vi "Calculate Counter And Protections.vi"(8 "error in (no error)":errorcluster, 9 "timeout ms":i32=100, 10 "Async Settings":T1={"Priority"=100, "CAN Session"="", "Frame Count"=0, "Frames"=[], "FPGA Session"=0, "Incoming Frame Session"="", "Incoming Session Invalid"=FALSE, "Incoming Frames"=[], "Signal Values"=[], "Incoming Signal Info"={"Signal.PrevData"=[], "Signal Names"=[], "Signal Settings Out"=[]}} {"Incoming Signal Info"."Signal Settings Out"."Protection Configuration"."CRC Channels"."Data Type" items=["Signed", "Unsigned", "IEEE Float"]; "Incoming Frames"."Protection Configurations"."CRC Channels"."Data Type" items=["Signed", "Unsigned", "IEEE Float"]; "Frames"."Protection Configurations"."CRC Channels"."Data Type" items=["Signed", "Unsigned", "IEEE Float"]}, 11 "Data Refs":T13) -> (0 "error out":errorcluster, 2 "Async Settings":T1={"Priority"=100, "CAN Session"="", "Frame Count"=0, "Frames"=[], "FPGA Session"=0, "Incoming Frame Session"="", "Incoming Session Invalid"=FALSE, "Incoming Frames"=[], "Signal Values"=[], "Incoming Signal Info"={"Signal.PrevData"=[], "Signal Names"=[], "Signal Settings Out"=[]}} {"Incoming Signal Info"."Signal Settings Out"."Protection Configuration"."CRC Channels"."Data Type" items=["Signed", "Unsigned", "IEEE Float"]; "Incoming Frames"."Protection Configurations"."CRC Channels"."Data Type" items=["Signed", "Unsigned", "IEEE Float"]; "Frames"."Protection Configurations"."CRC Channels"."Data Type" items=["Signed", "Unsigned", "IEEE Float"]})   [LabVIEW 2015, in "Protection and Counter Addon Engine.lvlib"]
uses:
  Protection and Counter Addon Engine.lvlib
  Types/RT Async Engine Variables.ctl
  SubModules/Frame Protection Support/Source/Engine/Types/RT Frame Settings.ctl
  SubModules/Frame Protection Support/Source/Shared/Types/Exported Frame Type.ctl
  SubModules/Frame Protection Support/Source/Engine/Types/RT Protection Configuration.ctl
  SubModules/Frame Protection Support/Source/Shared/Types/Protection Type.ctl
  SubModules/Frame Protection Support/Source/Shared/Types/XNET Signal Configuration.ctl
  SubModules/Frame Protection Support/Source/Shared/Types/Exported Counter Settings.ctl
  SubModules/Frame Protection Support/Source/Shared/Types/Exported Event Trigger Type.ctl
  SubModules/Frame Protection Support/Source/Shared/Types/Exported Frame Settings.ctl
  SubModules/Frame Protection Support/Source/Shared/Types/Exported Protection Settings.ctl
  SubModules/Frame Protection Support/Source/Shared/Types/RT_Incoming_Signal_Info.ctl
  SubModules/Frame Protection Support/Source/Shared/Types/RT Exported Signal Settings.ctl
  Types/RT Data References.ctl
  <vilib>/NI/NIVS Inline Async API/_Data Access Engine/Data Access Engine/Types/Write.DVR.ctl
  <vilib>/NI/NIVS Inline Async API/_Data Access Engine/Access Type Classes/Write/Write.lvclass
  <vilib>/NI/NIVS Inline Async API/_Data Access Engine/Data Access Engine/Types/Read.DVR.ctl
  <vilib>/NI/NIVS Inline Async API/_Data Access Engine/Access Type Classes/Read/Read.lvclass
  <vilib>/NI/NIVS Inline Async API/_Data Access Engine/Access Type Classes/Read/Read.lvclass/Read.ctl
  <vilib>/NI/NIVS Inline Async API/_Data Access Engine/Access Type Classes/Write/Write.lvclass/Write.ctl
  <vilib>/NI/NIVS Inline Async API/_Data Access Engine/Data Access Engine/Methods/Write.Data.vi
  <vilib>/NI/NIVS Inline Async API/_Data Access Engine/Access Type Classes/Write/Write.ProcessData.vi
  <vilib>/NI/NIVS Inline Async API/_Data Access Engine/Data Access Engine/Methods/Read.Data.Detect.vi
  <vilib>/NI/NIVS Inline Async API/_Data Access Engine/Data Access Engine/Methods/Write.Data.Buffer.vi
  SubModules/Frame Protection Support/Source/Engine/SubVIs/Determine Transmission.vi
  SubModules/Frame Protection Support/Source/Engine/SubVIs/Determine Periodic.vi
  <vilib>/NI/NIVS Inline Async API/_Data Access Engine/Data Access Engine/Methods/Write.Data.Commit.vi
  <vilib>/NI/NIVS Inline Async API/_Data Access Engine/Access Type Classes/Read/Read.ProcessData.Detect.vi
  <vilib>/NI/NIVS Inline Async API/_Data Access Engine/Access Type Classes/Write/Write.Buffer.vi
  <vilib>/NI/NIVS Inline Async API/_Data Access Engine/Access Type Classes/Write/Write.Commit.vi
  <vilib>/xnet/xnet.llb/XNET Write (Frame CAN).vi
  <vilib>/xnet/xnet.llb/XNET Convert.vi
  <vilib>/xnet/xnet.llb/XNET Convert (Signal to Frame CAN).vi
  <vilib>/xnet/xnet.llb/XNET Convert (Signal to Frame Raw).vi
  <vilib>/NI/NIVS Inline Async API/_Data Access Engine/Data Access Engine/Data Access Engine.lvclass
  SubModules/Frame Protection Support/Source/Engine/Protection and Counter Support Engine.lvlib
  SubModules/Frame Protection Support/Source/Shared/Protection and Counter Support Shared.lvlib
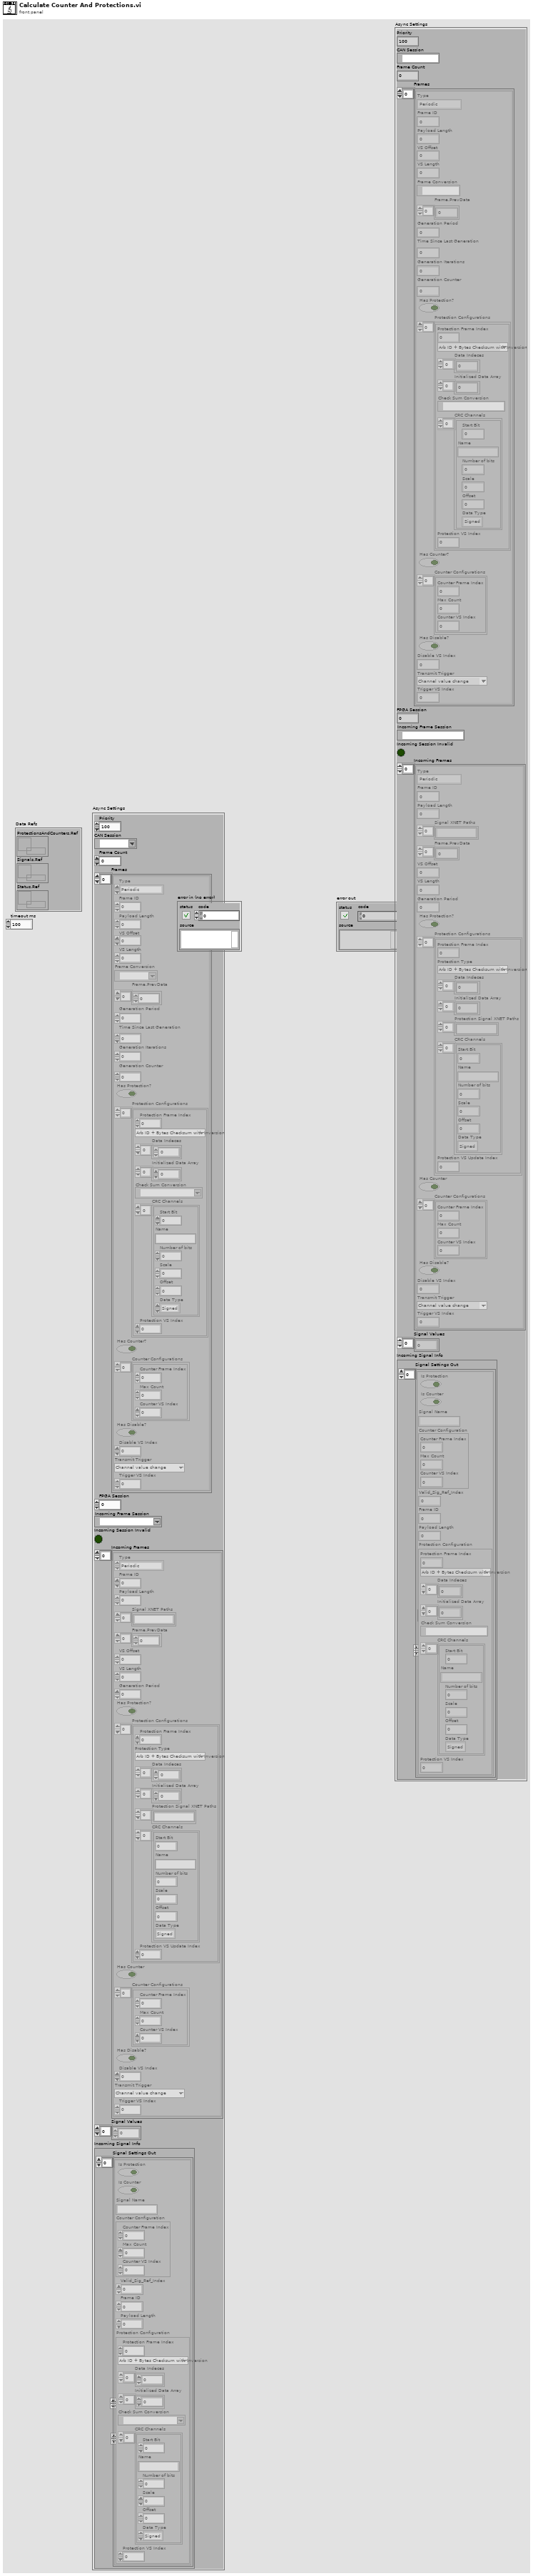
[diagram p1: front panel]
types:
  T1 = typedef "Protection and Counter Addon Engine.lvlib/RT Async Engine Variables.ctl" = cluster{"Priority":i32, "CAN Session":refnum<k21>, "Frame Count":i32, "Frames":T2[], "FPGA Session":u32, "Incoming Frame Session":refnum<k21>, "Incoming Session Invalid":bool, "Incoming Frames":T9[], "Signal Values":dbl[], "Incoming Signal Info":T11}
  T2 = typedef "Protection and Counter Support Engine.lvlib/RT Frame Settings.ctl" = cluster{"Type":T3, "Frame ID":u32, "Payload Length":u32, "VS Offset":i32, "VS Length":i32, "Frame Conversion":refnum<k21>, "Frame.PrevData":dbl[], "Generation Period":u32, "Time Since Last Generation":u32, "Generation Iterations":u32, "Generation Counter":u32, "Has Protection?":bool, "Protection Configurations":T4[], "Has Counter?":bool, "Counter Configurations":T7[], "Has Disable?":bool, "Disable VS Index":i32, "Transmit Trigger":T8, "Trigger VS Index":i32}
  T3 = typedef "Protection and Counter Support Shared.lvlib/Exported Frame Type.ctl" = enum16{"Periodic", "Event", "Periodic/Event"}
  T4 = typedef "Protection and Counter Support Engine.lvlib/RT Protection Configuration.ctl" = cluster{"Protection Frame Index":i32, "Protection Type":T5, "Data Indeces":i32[], "Initialized Data Array":dbl[], "Check Sum Conversion":refnum<k21>, "CRC Channels":T6[], "Protection VS Index":i32}
  T5 = typedef "Protection and Counter Support Shared.lvlib/Protection Type.ctl" = enum16{"Arb ID + Bytes Checksum with Inversion", "Arb ID + Bytes CRC with Inversion", "Reversed Raw Signal Checksum with Inversion"}
  T6 = typedef "Protection and Counter Support Shared.lvlib/XNET Signal Configuration.ctl" = cluster{"Start Bit":i32, "Name":string, "Number of bits":i32, "Scale":dbl, "Offset":dbl, "Data Type":u32}
  T7 = typedef "Protection and Counter Support Shared.lvlib/Exported Counter Settings.ctl" = cluster{"Counter Frame Index":i32, "Max Count":dbl, "Counter VS Index":i32}
  T8 = typedef "Protection and Counter Support Shared.lvlib/Exported Event Trigger Type.ctl" = enum16{"Channel value change", "Trigger channel (not zero)", "Channel value change or trigger channel (not zero)", "Trigger channel (any value change)", "Channel value change or trigger channel (any value change)"}
  T9 = typedef "Protection and Counter Support Shared.lvlib/Exported Frame Settings.ctl" = cluster{"Type":T3, "Frame ID":u32, "Payload Length":u32, "Signal XNET Paths":string[], "Frame.PrevData":dbl[], "VS Offset":i32, "VS Length":i32, "Generation Period":u32, "Has Protection?":bool, "Protection Configurations":T10[], "Has Counter":bool, "Counter Configurations":T7[], "Has Disable?":bool, "Disable VS Index":i32, "Transmit Trigger":T8, "Trigger VS Index":i32}
  T10 = typedef "Protection and Counter Support Shared.lvlib/Exported Protection Settings.ctl" = cluster{"Protection Frame Index":i32, "Protection Type":T5, "Data Indeces":i32[], "Initialized Data Array":dbl[], "Protection Signal XNET Paths":string[], "CRC Channels":T6[], "Protection VS Update Index":i32}
  T11 = typedef "Protection and Counter Support Shared.lvlib/RT_Incoming_Signal_Info.ctl" = cluster{"Signal.PrevData":dbl[], "Signal Names":string[], "Signal Settings Out":T12[]}
  T12 = typedef "Protection and Counter Support Shared.lvlib/RT Exported Signal Settings.ctl" = cluster{"Is Protection":bool, "Is Counter":bool, "Signal Name":string, "Counter Configuration":T7, "Valid_Sig_Ref_Index":i32, "Frame ID":u32, "Payload Length":u32, "Protection Configuration":T4}
  T13 = typedef "Protection and Counter Addon Engine.lvlib/RT Data References.ctl" = cluster{"ProtectionsAndCounters.Ref":T14, "Signals.Ref":T15, "Status.Ref":T14}
  T14 = typedef "Data Access Engine.lvlib/Data Access Engine.lvclass/Write.DVR.ctl" = refnum<data-value>
  T15 = typedef "Data Access Engine.lvlib/Data Access Engine.lvclass/Read.DVR.ctl" = refnum<data-value>
  T16 = typedef "XNET Frame CAN.ctl" = cluster{"timestamp":timestamp, "payload":u8[], "identifier":u32, "type":T17, "extended?":bool, "echo?":bool}
  T17 = typedef "XNET Frame Type CAN.ctl" = u8
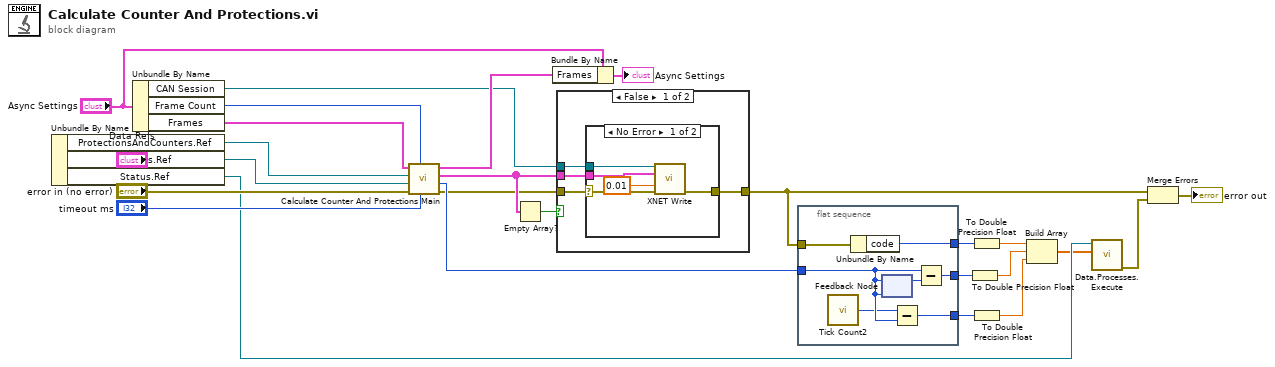
[diagram p0: block diagram]
diagram:
  n1 = Unbundle By Name("Data Refs") -> ("ProtectionsAndCounters.Ref"=w1:T14, "Signals.Ref"=w21:T15, "Status.Ref"=w19:T14)
  n2 = Unbundle By Name("Async Settings") -> ("CAN Session"=w6:refnum<k21>, "Frame Count"=w23:i32, "Frames"=w2:T2[])
  n3 = call "Calculate Counter And Protections Main.vi"("timeout ms"="timeout ms", "Frame Count"=w23, "error in (no error)"="error in (no error)", "Signals"=w21, "Protections"=w1, "Frames in"=w2) -> ("error out"=w5:errorcluster, "Tick Count(uSec)"=w20:u32, "Frames"=w9:T16[], "Frames out"=w11:T2[])  [unwired: 2 in]
  n4 = Empty Array?(array=w9) -> (empty?=w8:bool)
  n5 = Bundle By Name(cluster="Async Settings", "Frames"=w11) -> (→"Async Settings":T1)
  n6 = case shown="False" w8 {
    tunnel: w5 -> [w30 w37]
    tunnel: [w29 w37] -> w4
    tunnel: w6 -> [w28 _]
    tunnel: w9 -> [w27 _]
    frame False {
      n7 = case shown="No Error" w30 {
        selector: w30 -> [w32 w36]
        tunnel: w27 -> [w35 _]
        tunnel: [w34 w36] -> w29
        tunnel: w28 -> [w33 _]
        frame No Error {
          n8 = call-poly <vilib>:"XNET Write.vi"("session in"=w33, "data"=w35, "timeout (10)"=0.01, "error in (no error)"=w32) -> ("error out"=w34:errorcluster)  [unwired: 10 in, 1 out]
        }
        frame Error {
        }
      }
    }
    frame True {
    }
  }
  n9 = flat-sequence {
    tunnel: w20 -> [w44]
    tunnel: [w43] -> w18
    tunnel: [w42] -> w15
    tunnel: w4 -> [w39]
    tunnel: [w38] -> w7
    frame #0 {
      n10 = call "Tick Count2"() -> ("Tick Count(uSec)"=w41:u32)
      n11 = Unbundle By Name(w39) -> ("code"=w38:i32)
      n12 = feedback #1(w44) -> (w40:u32)
      n13 = feedback-in #1(w44) -> ()
      n14 = Subtract(x=w41, y=w44) -> (x-y=w42:u32)
      n15 = Subtract(x=w44, y=w40) -> (x-y=w43:u32)
    }
  }
  n16 = To Double Precision Float(number=w18) -> (double precision float=w13:dbl)
  n17 = To Double Precision Float(number=w7) -> (double precision float=w14:dbl)
  n18 = To Double Precision Float(number=w15) -> (double precision float=w12:dbl)
  n19 = Build Array(w14, w13, w12) -> (w17:dbl[])
  n20 = call-poly <vilib>:"Data.Processes.Execute.vi"("Values"=w17, "Ref"=w19) -> ("error out"=w16:errorcluster)  [unwired: 9 in]
  n21 = Merge Errors(w4, w16) -> (→"error out":errorcluster)
